vi "SaveMessage.vi"() -> ()   [LabVIEW 2017]
uses:
  SaveMessage.ctl
panel:
  in  "Save message":T1
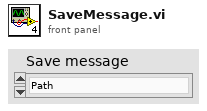
[diagram p1: front panel]
types:
  T1 = typedef "SaveMessage.ctl" = enum16{"Path", "StartSaving", "StopSaving", "Ch1Value", "Ch2Value", "Ch3Value"}
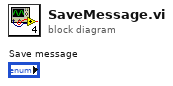
[diagram p0: block diagram]
diagram:
